vi "ge_CloseAllQs.vi"(8 "error in":errorcluster) -> (0 "error out":errorcluster)   [LabVIEW 2012]
uses:
  Custom Ctrls/ge_AMC_Qname.ctl
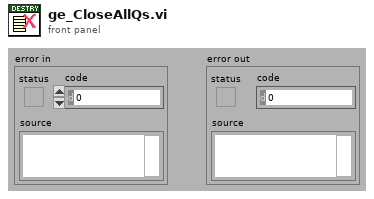
[diagram p1: front panel]
types:
  T1 = typedef "ge_AMC_Qname.ctl" = enum16{"Cmnd Loop", "UI Updater", "Conn Mgr HS", "Conn Mgr LS", "TCP Send HS", "TCP Send LS"}
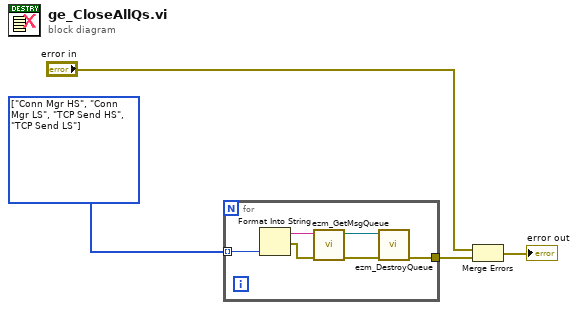
[diagram p0: block diagram]
diagram:
  w4 = T1[] [enum."Conn Mgr HS", enum."Conn Mgr LS", enum."TCP Send HS", enum."TCP Send LS"] items=["Cmnd Loop", "UI Updater", "Conn Mgr HS", "Conn Mgr LS", "TCP Send HS", "TCP Send LS"]
  n1 = for {
    tunnel: [w8] -> w3
    tunnel: w4 -> [w6] mode=indexing
    n2 = Format Into String(w6) -> (resulting string=w5:string, error out=w7:errorcluster)  [unwired: 3 in]
    n3 = call "ezm_GetMsgQueue.vi"("error in"=w7, "Queue Name"=w5) -> ("error out"=w9:errorcluster, "queue out"=w10:refnum<queue>)  [unwired: 8 in]
    n4 = call "ezm_DestroyQueue.vi"("error in (no error)"=w9, "Queue in"=w10) -> ("error out"=w8:errorcluster)  [unwired: 9 in]
  }
  n5 = Merge Errors("error in", w3) -> (→"error out":errorcluster)
